vi "Sandbox.vi"() -> ()   [LabVIEW 2018]
uses:
  support/classes/Category/Category.lvclass
  support/classes/database/Account History.lvclass
panel:
  out "Category.lvclass":refnum<class "Category.lvclass">
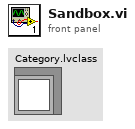
[diagram p1: front panel]
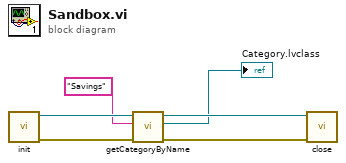
[diagram p0: block diagram]
diagram:
  n1 = call "init.vi"() -> ("error out"=w4:errorcluster, "Database.lvclass"=w6:refnum<class "Account History.lvclass">)  [unwired: 10 in]
  n2 = call "getCategoryByName.vi"("error in (no error)"=w4, "Name"="Savings", "Account History in"=w6) -> ("error out"=w3:errorcluster, "Category.lvclass"=→"Category.lvclass":refnum<class "Category.lvclass">, "Account History out"=w5:refnum<class "Account History.lvclass">)  [unwired: 6 in]
  n3 = call "close.vi"("error in (no error)"=w3, "Database.lvclass"=w5) -> ()  [unwired: 9 in, 1 out]
